vi "CalculateDeltas_v5.vi"(0 "Method":T1(ring), 1 "Which Order?":enum16{"No Calculation", "Ref-Sam", "Sam-Ref"}(ring), 2 "Input 2D Numeric Array":dbl[][](array[numeric])) -> (4 "Array - Ratio Sam/Ref":dbl[][](array[numeric]), 5 "Number of Comparisons":i32, 6 "Array - Ref Rows":dbl[][](array[numeric]), 7 "Array - Sample Rows":dbl[][](array[numeric]), 8 "Column-wise Mean of Ratios":dbl[](array[numeric]), 9 "Column-wise STDEVs of Ratios":dbl[](array[numeric]))   [LabVIEW 2013]
doc: "This VI takes as input a 2D numeric array consisting of Running Output from TDLWintel (RS-232 stream), and calculates difference (ratio) between Sample and Reference Rows. \n\nOther inputs are \"Method\" (currently only Bellow1-Bellow2 or Recycle are available), and (for Bellow to Bellow comparison method only) the Bellow to be used as Reference."
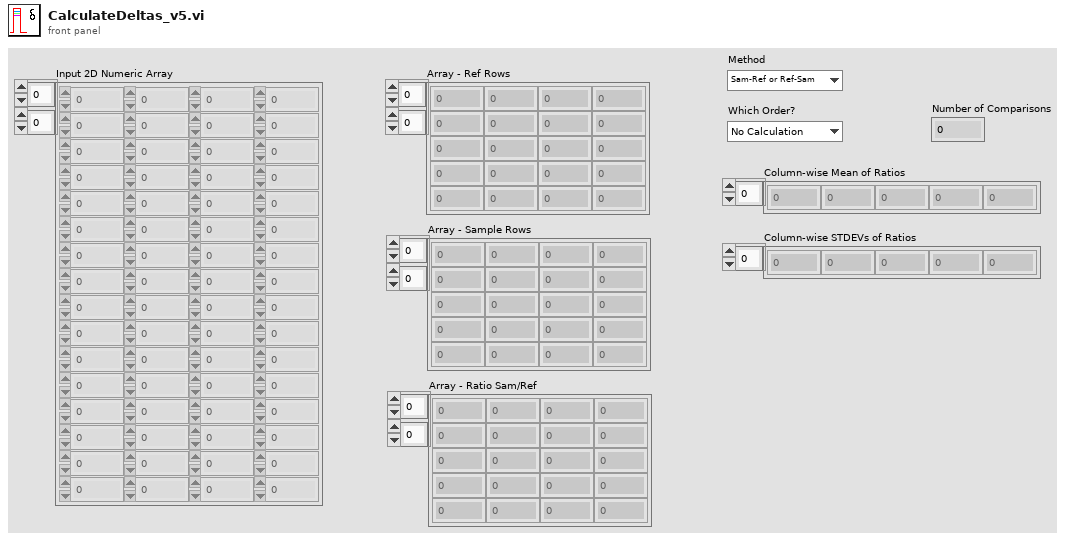
[diagram p1: front panel]
types:
  T1 = enum16{"Sam-Ref or Ref-Sam", "Recycle (Ref-Sam-Ref)"}
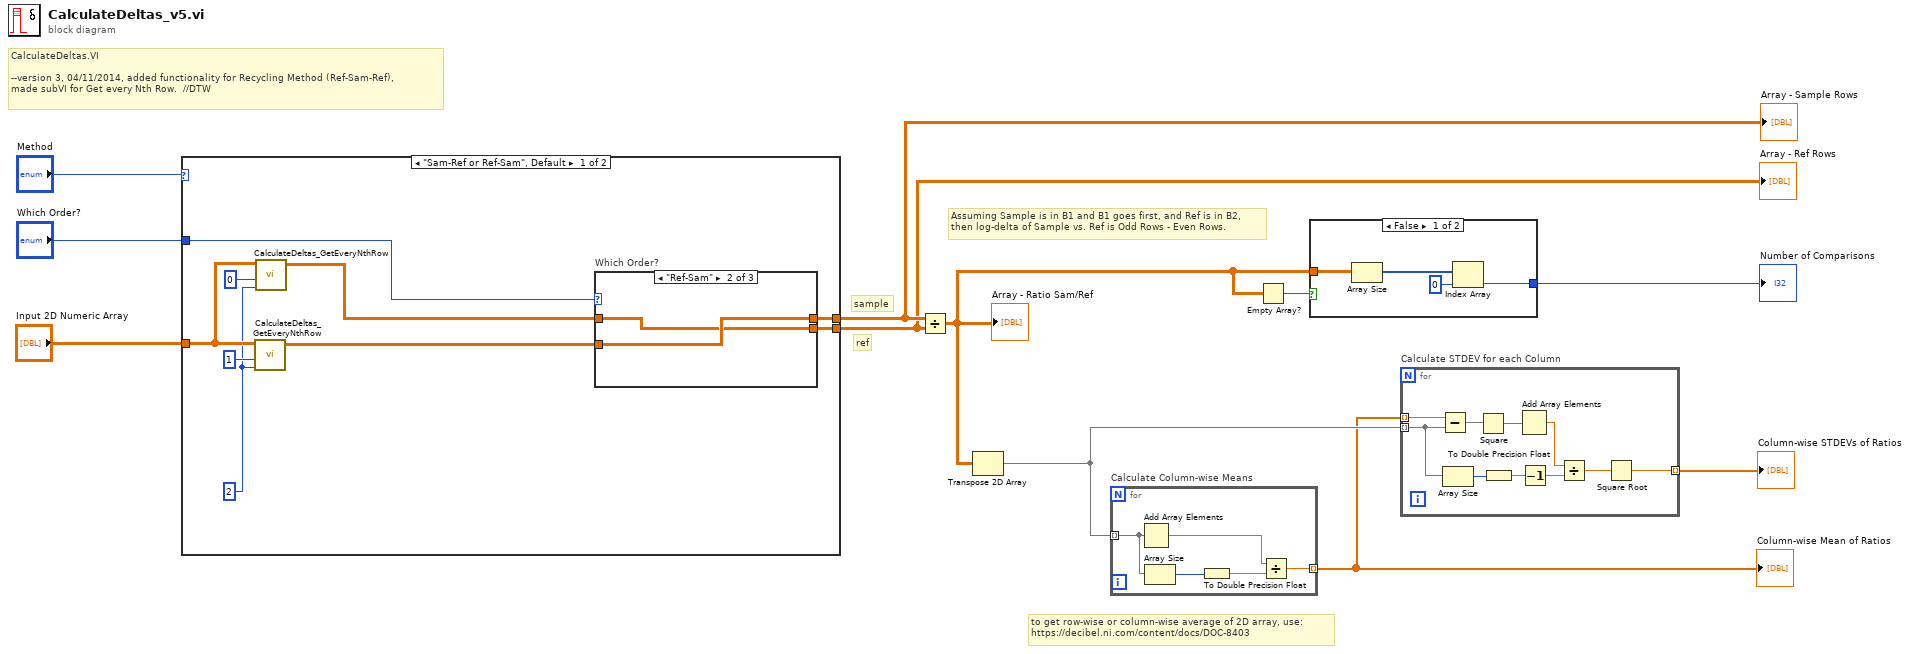
[diagram p0: block diagram]
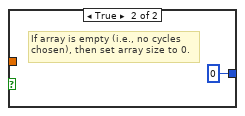
[diagram p2: hidden frame]
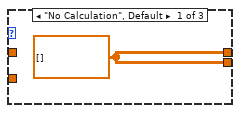
[diagram p3: hidden frame]
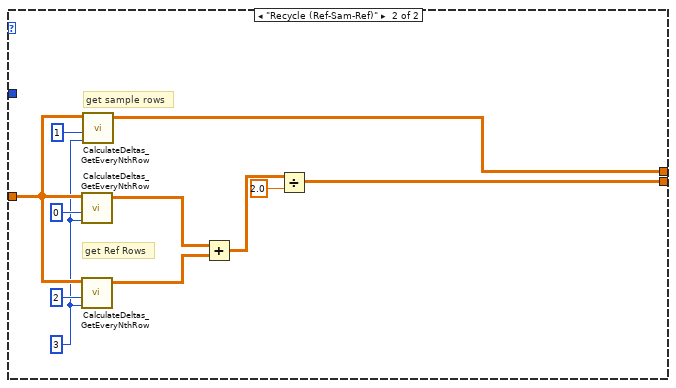
[diagram p5: hidden frame]
diagram:
  # "ref"
  # "CalculateDeltas.VI\n\n--version 3, 04/11/2014, added functionality for Recycling Method (Ref-Sam-Ref), \nmade subVI for Get every Nth Row.  //DTW"
  # "sample"
  # "to get row-wise or column-wise average of 2D array, use: \nhttps://decibel.ni.com/content/docs/DOC-8403"
  # "Assuming Sample is in B1 and B1 goes first, and Ref is in B2,\nthen log-delta of Sample vs. Ref is Odd Rows - Even Rows."
  n1 = case shown="\"Sam-Ref or Ref-Sam\", Default" "Method" {
    tunnel: "Input 2D Numeric Array" -> [w13 w33]
    tunnel: "Which Order?" -> [w20 _]
    tunnel: [w18 w26] -> w6
    tunnel: [w17 w29] -> w5
    frame "Sam-Ref or Ref-Sam", Default {
      w12 = 2 ("Get every n-th Row:")
      n2 = call "CalculateDeltas_GetEveryNthRow.vi"("Input 2D Numeric Array"=w13, "First Row's Index"=1, "Get every n-th Row:"=w12) -> ("Output Rows"=w14:dbl[][])  [unwired: 5 in]
      n3 = call "CalculateDeltas_GetEveryNthRow.vi"("Input 2D Numeric Array"=w13, "First Row's Index"=0, "Get every n-th Row:"=w12) -> ("Output Rows"=w19:dbl[][])  [unwired: 5 in]
      n4 = case "Which Order?" shown="\"Ref-Sam\"" w20 {
        tunnel: w19 -> [_ w22 w25]
        tunnel: [w21 w23 w25] -> w18
        tunnel: [w21 w22 w24] -> w17
        tunnel: w14 -> [_ w23 w24]
        frame "No Calculation", Default {
          w21 = dbl[][] []
        }
        frame "Ref-Sam" {
        }
        frame "Sam-Ref" {
        }
      }
    }
    frame "Recycle (Ref-Sam-Ref)" {
      w32 = 3 ("Get every n-th Row:")
      # "get Ref Rows"
      # "get sample rows"
      n5 = call "CalculateDeltas_GetEveryNthRow.vi"("Input 2D Numeric Array"=w33, "First Row's Index"=0, "Get every n-th Row:"=w32) -> ("Output Rows"=w31:dbl[][])  [unwired: 5 in]
      n6 = call "CalculateDeltas_GetEveryNthRow.vi"("Input 2D Numeric Array"=w33, "First Row's Index"=2, "Get every n-th Row:"=w32) -> ("Output Rows"=w30:dbl[][])  [unwired: 5 in]
      n7 = call "CalculateDeltas_GetEveryNthRow.vi"("Input 2D Numeric Array"=w33, "First Row's Index"=1, "Get every n-th Row:"=w32) -> ("Output Rows"=w26:dbl[][])  [unwired: 5 in]
      n8 = Add(x=w31, y=w30) -> (x+y=w27:dbl[][])
      n9 = Divide(x=w27, y=2.0) -> (x/y=w29:dbl[][])
    }
  }
  "Array - Sample Rows" <- w6
  "Array - Ref Rows" <- w5
  n10 = Divide(x=w6, y=w5) -> (x/y=w1:dbl[][])
  "Array - Ratio Sam/Ref" <- w1
  n11 = Transpose 2D Array(2D array=w1) -> (transposed array=w10:dbl[][])
  n12 = for "Calculate Column-wise Means" {
    tunnel: w10 -> [w39] mode=indexing
    tunnel: [w40] -> w3 mode=indexing
    n13 = Add Array Elements(numeric array=w39) -> (sum=w41:dbl)
    n14 = Array Size(array=w39) -> (size(s)=w38:i32)
    n15 = To Double Precision Float(number=w38) -> (double precision float=w37:dbl)
    n16 = Divide(x=w41, y=w37) -> (x/y=w40:dbl)
  }
  "Column-wise Mean of Ratios" <- w3
  n17 = Empty Array?(array=w1) -> (empty?=w2:bool)
  n18 = case shown="False" w2 {
    tunnel: [w43 0] -> w8
    tunnel: w1 -> [w42 _]
    frame False {
      n19 = Array Size(array=w42) -> (size(s)=w45:i32[])
      n20 = Index Array "Index Array"(array=w45, index=0) -> (element=w43:i32)
    }
    frame True {
      # "If array is empty (i.e., no cycles\nchosen), then set array size to 0."
    }
  }
  "Number of Comparisons" <- w8
  n21 = for "Calculate STDEV for each Column" {
    tunnel: w10 -> [w50] mode=indexing
    tunnel: [w48] -> w11 mode=indexing
    tunnel: w3 -> [w47] mode=indexing
    n22 = Subtract(x=w47, y=w50) -> (x-y=w56:dbl[])
    n23 = Array Size(array=w50) -> (size(s)=w51:i32)
    n24 = Square(x=w56) -> (x^2=w55:dbl[])
    n25 = To Double Precision Float(number=w51) -> (double precision float=w53:dbl)
    n26 = Add Array Elements(numeric array=w55) -> (sum=w54:dbl)
    n27 = Decrement(x=w53) -> (x-1=w52:dbl)
    n28 = Divide(x=w54, y=w52) -> (x/y=w49:dbl)
    n29 = Square Root(x=w49) -> (sqrt(x)=w48:dbl)
  }
  "Column-wise STDEVs of Ratios" <- w11
